vi "load and intialize target with engines.vi"(6 "timeout in ms (-1)":i32=-1, 8 "error in":errorcluster, 9 "engine aliases (empty = ALL)":string[](array[string]), 10 "target alias":string, 11 "file path":path) -> (0 "error out":errorcluster, 2 "engine runtime interfaces":refnum<class "Engine Runtime Interface.lvclass">[](array[class]), 3 "target runtime":refnum<class "PL_Target Runtime.lvclass">)   [LabVIEW 2014, in "PL_Target Runtime.lvclass"]
doc: "Loads and initializes the target specified by 'target alias' for the configuration file specified by 'file path'. This VI returns an initialized target object with an array of engine objects which can be interacted with using the Engine Execution Interface APIs."
uses:
  PL_Target Runtime.lvclass
  <vilib>/NI/Module Execution Interface/Engine Runtime/Engine Runtime Interface.lvclass
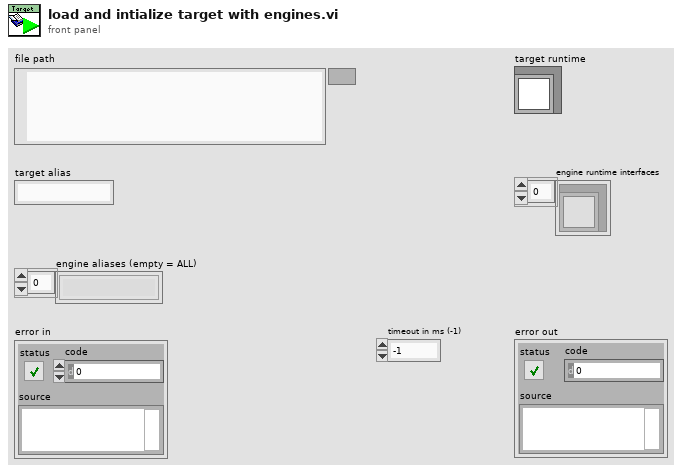
[diagram p1: front panel]
types:
  T1 = typedef "PLConfigurationSerializer.lvlib/engines cluster.ctl" = cluster{"engine configuration":refnum<class "engine configuration.lvclass">, "modules":refnum<class "TBM module configuration.lvclass">[]}
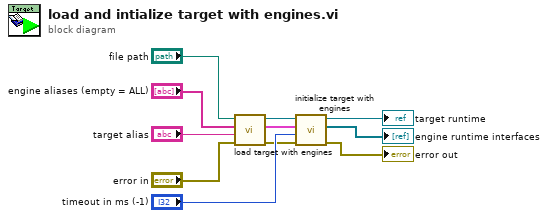
[diagram p0: block diagram]
diagram:
  n1 = call "load target with engines.vi"("error in (no error)"="error in", "target alias"="target alias", "engine aliases (empty = ALL)"="engine aliases (empty = ALL)", "file path"="file path") -> ("error out"=w3:errorcluster, "engines"=w1:T1[], "PL_Target Configuration out"=w2:refnum<class "PL_Target Configuration.lvclass">)  [unwired: 5 in]
  n2 = call "initialize target with engines.vi"("error in (no error)"=w3, "timeout in ms (-1)"="timeout in ms (-1)", "engines"=w1, "PL_Target Configuration in"=w2) -> ("error out"=→"error out":errorcluster, "Array"=→"engine runtime interfaces":refnum<class "Engine Runtime Interface.lvclass">[], "PL_Target Runtime out"=→"target runtime":refnum<class "PL_Target Runtime.lvclass">)  [unwired: 5 in]
